vi "Close MeasurementLink Session.vi"(8 "error in":errorcluster, 9 "initialize and close session behavior":T1, 10 "session in":variant, 11 "session factory in":refnum<class "Session Factory.lvclass">) -> (0 "error out":errorcluster)   [LabVIEW 2021, in "NI Session Management niSwitch.lvlib" / "Session Factory.lvclass"]
doc: "Closes the local session. If the session represents a remote session, <b>initialize and close session behavior</b> determines whether closing the local session closes the server session or detaches from the server session."
uses:
  Session Factory.lvclass
  <vilib>/Plug-In SDKs/Sessions/Instrument/ISession Factory/Initialize and Close Session Behavior.ctl
  Session Factory.lvclass/Session Factory.ctl
  NI Switch_client/RPC Messages/niswitch_grpc_CloseRequest.ctl
  NI Switch_client/RPC Messages/nidevice_grpc_Session.ctl
  NI Switch_client/RPC Messages/nidevice_grpc_Session_session/nidevice_grpc_Session_session.lvclass
  NI Switch_client/NI Switch_client.lvlib
  <vilib>/Plug-In SDKs/Sessions/Instrument/ISession Factory/ISession Factory.lvclass
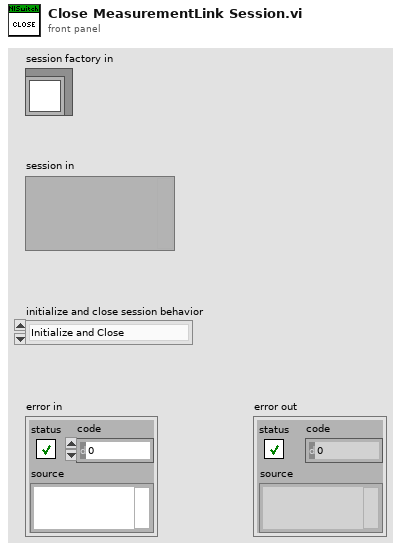
[diagram p1: front panel]
types:
  T1 = typedef "NI Session Management Instrument.lvlib/ISession Factory.lvclass/Initialize and Close Session Behavior.ctl" = enum16{"Initialize and Close", "Attach and Detach", "Initialize and Detach", "Attach and Close"}
  T2 = typedef "NI Switch_client.lvlib/niswitch_grpc_CloseRequest.ctl" = cluster{"vi":T3}
  T3 = typedef "NI Switch_client.lvlib/nidevice_grpc_Session.ctl" = cluster{"nidevice_grpc_Session_session":refnum<class "nidevice_grpc_Session_session.lvclass">}
  T4 = typedef "grpc-lvsupport-release.lvlib/grpcId.ctl" = u64
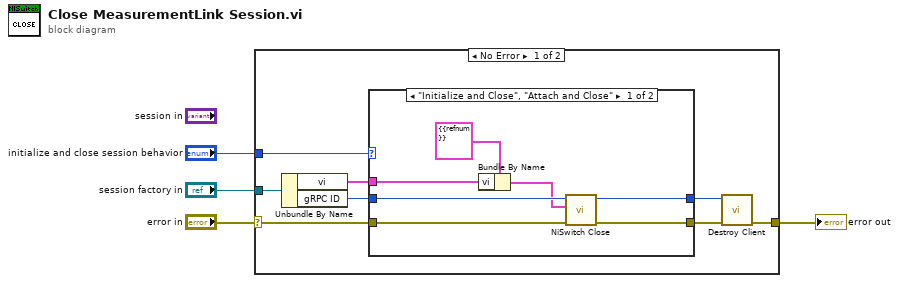
[diagram p0: block diagram]
diagram:
  n1 = case shown="No Error" "error in" {
    selector: "error in" -> [w12 w22]
    tunnel: [w10 w22] -> w4
    tunnel: "initialize and close session behavior" -> [w9 _]
    tunnel: "session factory in" -> [w6 _]
    frame No Error {
      n2 = Unbundle By Name(w6) -> ("vi"=w7:T3, "gRPC ID"=w8:T4)
      n3 = case shown="\"Initialize and Close\", \"Attach and Close\"" w9 {
        tunnel: w12 -> [w19 w21]
        tunnel: [w18 w21] -> w11
        tunnel: w8 -> [w15 w20]
        tunnel: [w17 w20] -> w5
        tunnel: w7 -> [w13 _]
        frame "Initialize and Close", "Attach and Close" {
          n4 = Bundle By Name(cluster=T2 {"vi"={"nidevice_grpc_Session_session"=refnum}} ("Request Data"), "vi"=w13) -> (w14:T2)
          n5 = call "NiSwitch Close.vi"("error in"=w19, "Request Data"=w14, "gRPC ID"=w15) -> ("error out"=w18:errorcluster, "gRPC ID out"=w17:T4)  [unwired: 6 in, 1 out]
        }
        frame "Attach and Detach", "Initialize and Detach" {
        }
      }
      n6 = call "Destroy Client.vi"("error in"=w11, "gRPC ID"=w5) -> ("error out"=w10:errorcluster)  [unwired: 9 in]
    }
    frame Error {
    }
  }
  "error out" <- w4
